vi "Handle Asynchronous.vi"(8 "error in (no error)":errorcluster, 9 "Message Data":variant, 10 "Message":string, 11 "Asynchronous Action In":refnum<class "Async Handler.lvclass">) -> (0 "error out":errorcluster, 3 "Asynchronous Action Out":refnum<class "Async Handler.lvclass">)   [LabVIEW 2020, in "Async Handler.lvclass"]
doc: "The specific action implemented in the asynchronous action. Multiple different actions may be supported by using the Message and Message Data input to separate them. Any number of actions may run in parallell running the same or different actions. If this method throws an error, the error will be sent to the error handler configured for the process. \nCare needs to be taken so that this action is cancelled if the process is stopped. This may be detected by e.g. observing the Lifecycle: Stopped/Finished broadcast or polling the Get Lifecycle State.vi."
uses:
  Async Handler.lvclass
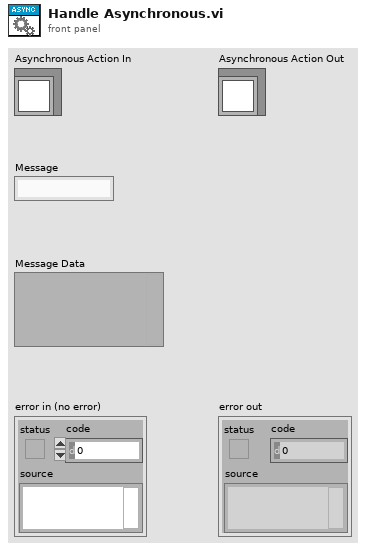
[diagram p1: front panel]
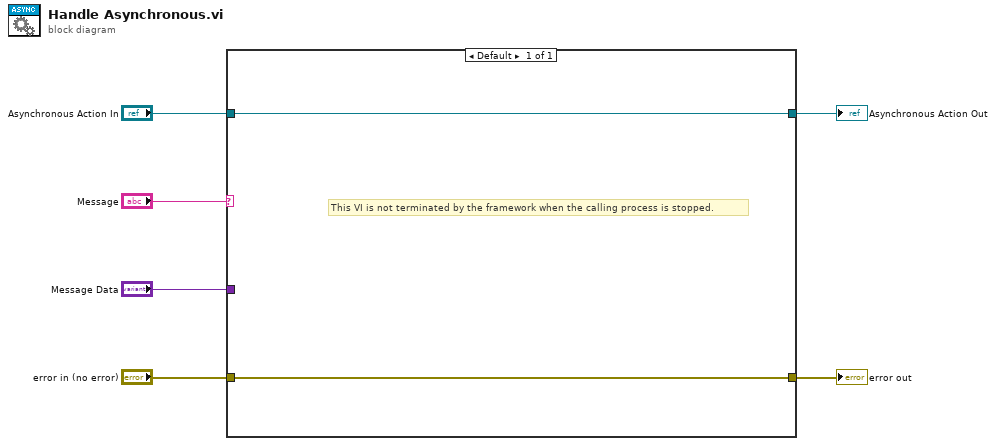
[diagram p0: block diagram]
diagram:
  n1 = case shown="Default" "Message" {
    tunnel: [w8] -> w6
    tunnel: "Asynchronous Action In" -> [w8]
    tunnel: [w7] -> w4
    tunnel: "error in (no error)" -> [w7]
    tunnel: "Message Data" -> [_]
    frame Default {
      # "This VI is not terminated by the framework when the calling process is stopped."
    }
  }
  "error out" <- w4
  "Asynchronous Action Out" <- w6
